vi "Get In User Documents.vi"(10 "error in (no error)":errorcluster) -> (2 "error out":errorcluster, 3 "Base In User Documents":path)   [LabVIEW 2021, in "Path Utilities.lvlib"]
doc: "Returns User Documents path appended with base path.\neg: \"C:\\Users\\Name\\Documents\\Base\\Path\""
uses:
  Path Utilities.lvlib
  TypeDefs/FGV State.ctl
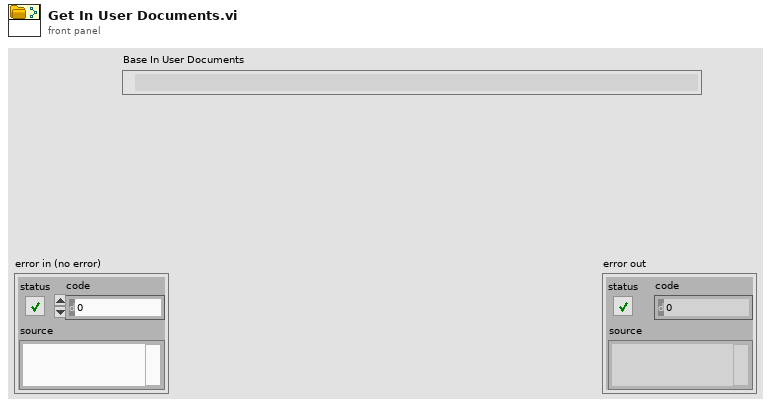
[diagram p1: front panel]
types:
  T1 = typedef "Path Utilities.lvlib/FGV State.ctl" = enum16{"Set Base Path", "Get Program Files", "Get Program Data", "Get App Data Local", "Get App Data Roaming", "Get User Documents", "Get Public Documents"}
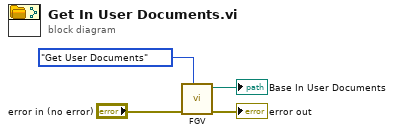
[diagram p0: block diagram]
diagram:
  n1 = call "FGV.vi"("FGV State"=FGV_State."Get User Documents", "error in (no error)"="error in (no error)") -> ("error out"=→"error out":errorcluster, "Path Out"=→"Base In User Documents":path)  [unwired: 8 in]
